vi "Is DateTime String.vi"(11 "string or date/time":variant) -> (1 "database data type":T1, 3 "data":string)   [LabVIEW 2011]
uses:
  <vilib>/addons/database/Auxilliary.llb/DB Tools DataTypes.ctl
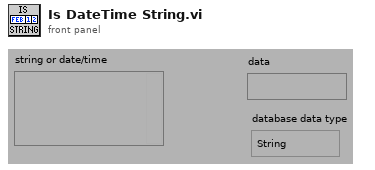
[diagram p1: front panel]
types:
  T1 = typedef "NI_Database_API.lvlib/DB Tools DataTypes.ctl" = enum16{"String", "Long (I32)", "Single (SGL)", "Double (DBL)", "Date/Time", "Binary"}
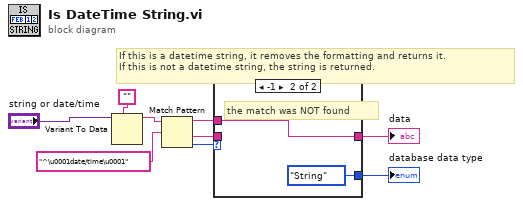
[diagram p0: block diagram]
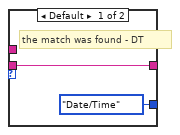
[diagram p2: hidden frame]
diagram:
  # "If this is a datetime string, it removes the formatting and returns it.  \nIf this is not a datetime string, the string is returned."
  n1 = Variant To Data(type="", Variant="string or date/time") -> (data=w3:string)  [unwired: 1 in, 1 out]
  n2 = Match Pattern(string=w3, regular expression="^\u0001date/time\u0001" ("string (\"\")")) -> (before substring=w6:string, after substring=w5:string, offset past match=w9:i32)  [unwired: 1 in, 1 out]
  n3 = case shown="-1" w9 {
    tunnel: w5 -> [w11 _]
    tunnel: w6 -> [_ w13]
    tunnel: [w11 w13] -> w7
    tunnel: [DB_Tools_DataTypes."Date/Time" ("database data type") DB_Tools_DataTypes."String" ("database data type")] -> w8
    frame Default {
      # "the match was found - DT"
    }
    frame -1 {
      # "the match was NOT found"
    }
  }
  "data" <- w7
  "database data type" <- w8
